vi "OAT Torsional Vibration (Digital Tacho) (Waveform) (1 Ch).vi"(0 "digital tacho info":T1={"tacho counts"=[], "counter timebase [Hz]"=1000.0, "counter task type"=enum."event counting", "counter digit (32)"=32}, 2 "pulse/revolution (1)":i32=1 min=1, 4 "torsional vibration units":enum16{"RPM", "deg/s", "rad/s"}(ring), 5 "error in (no error)":errorcluster, 8 "reset? (F)":bool, 10 "compensate geometric imperfection? (F)":bool, 11 "output interval [s]":dbl=0.001 min=0.0) -> (14 "torsional vibration signal":waveform(dbl), 15 "speed profile":T2 {"speed [RPM]" format="%.2f"; "time [s]" format="%.2f"}, 18 "unit label":string, 19 "error out":errorcluster)   [LabVIEW 2017, in "SoundVib_Torsional.lvlib"]
doc: "Calculates torsional vibration signals from digital tachometer signals. This VI can return torsional vibration signals as either waveform signals or even-angle signals. Wire data to the <B>digital tacho info</B> input to determine the polymorphic instance to use or manually select the instance."
uses:
  <vilib>/addons/Sound and Vibration/Order Analysis/Torsional Vibration/SoundVib_Torsional.lvlib
  <vilib>/addons/Sound and Vibration/Order Analysis/Tach Process/SubVIs/speed profile.ctl
  <vilib>/addons/Sound and Vibration/Order Analysis/Tach Process/SubVIs/digital tach info.ctl
  <vilib>/addons/Sound and Vibration/Order Analysis/Tach Process/SoundVib_TachProcess.lvlib
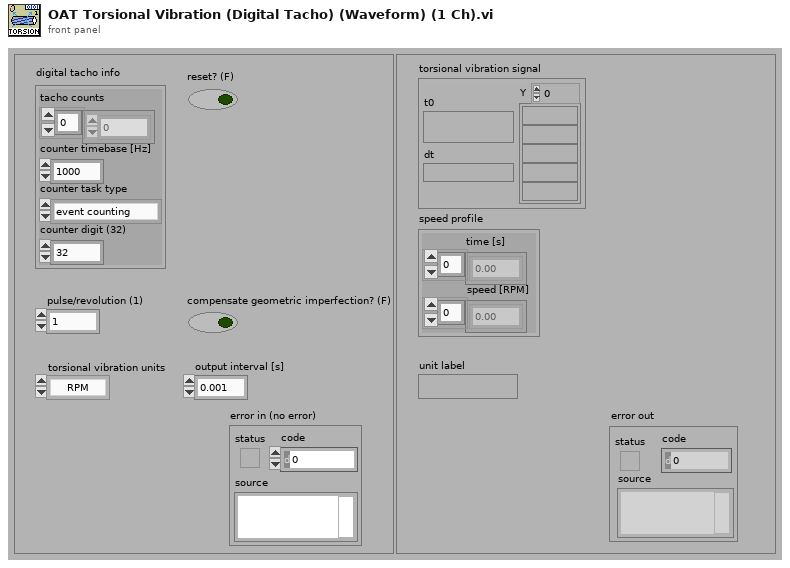
[diagram p1: front panel]
types:
  T1 = typedef "SoundVib_TachProcess.lvlib/digital tach info.ctl" = cluster{"tacho counts":i64[], "counter timebase [Hz]":dbl, "counter task type":enum16{"period measurement", "event counting"}, "counter digit (32)":i32}
  T2 = typedef "SoundVib_TachProcess.lvlib/speed profile.ctl" = cluster{"time [s]":dbl[], "speed [RPM]":dbl[]}
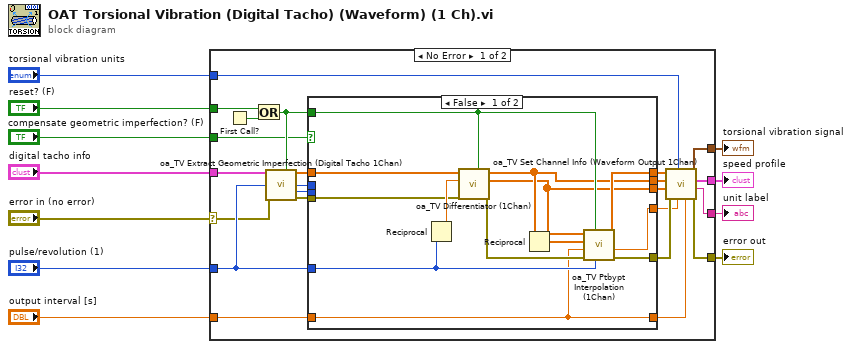
[diagram p0: block diagram]
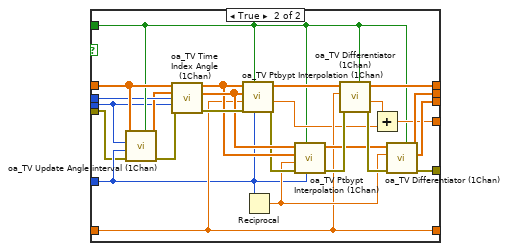
[diagram p2: hidden frame]
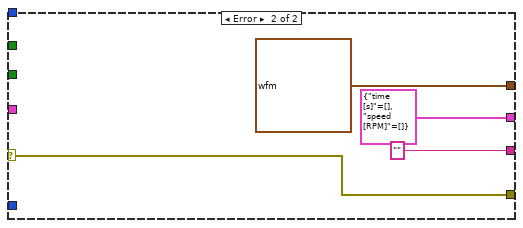
[diagram p3: hidden frame]
diagram:
  n1 = case shown="No Error" "error in (no error)" {
    selector: "error in (no error)" -> [w25 w75]
    tunnel: "pulse/revolution (1)" -> [w27 _]
    tunnel: [w20 waveform(dbl) {"t0"=timestamp(0 s since 1904-01-01), "dt"=1.0, "Y"=[]} ("even time speed")] -> w11
    tunnel: "compensate geometric imperfection? (F)" -> [w13 _]
    tunnel: "reset? (F)" -> [w31 _]
    tunnel: "digital tacho info" -> [w29 _]
    tunnel: "output interval [s]" -> [w18 _]
    tunnel: "torsional vibration units" -> [w19 _]
    tunnel: [w23 w75] -> w5
    tunnel: [w16 T2 {"time [s]"=[], "speed [RPM]"=[]} ("speed profile")] -> w4
    tunnel: [w12 "" ("unit label")] -> w1
    frame No Error {
      n2 = First Call?() -> (First Call?: T/F=w32:bool)
      n3 = Or(x=w31, y=w32) -> (x .or. y?=w26:bool)
      n4 = call <vilib>:"oa_TV Extract Geometric Imperfection (Digital Tacho 1Chan).vi"("digital tach info"=w29, "reset? (F)"=w26, "pulse/revolution"=w27, "error in (no error)"=w25) -> ("pulse positions"=w28:dbl[], "revulotion"=w30:i32, "revulotion index"=w33:i32, "error out"=w34:errorcluster)  [unwired: 8 in]
      n5 = case shown="False" w13 {
        tunnel: w34 -> [w45 w49]
        tunnel: w33 -> [_ w51]
        tunnel: w30 -> [_ w53]
        tunnel: w28 -> [w47 w55]
        tunnel: w27 -> [w43 w50]
        tunnel: w26 -> [w39 w54]
        tunnel: [w35 w65] -> w24
        tunnel: [w38 w64] -> w22
        tunnel: [w44 w63] -> w21
        tunnel: w18 -> [w41 w59]
        tunnel: [w36 w56] -> w17
        tunnel: [w37 w60] -> w15
        tunnel: [w41 w59] -> w14
        frame False {
          n6 = Reciprocal(x=w43) -> (1/x=w46:dbl)
          n7 = call <vilib>:"oa_TV Differentiator (1Chan).vi"("reset? (True)"=w39, "error in (no error)"=w45, "deltaX"=w46, "Y[n]"=w47) -> ("error out"=w42:errorcluster, "X[n]"=w37:dbl[], "dY[n]/dX[n]"=w38:dbl[])  [unwired: 4 in, 1 out]
          n8 = Reciprocal(x=w38) -> (1/x=w40:dbl[])
          n9 = call <vilib>:"oa_TV Ptbypt Interpolation (1Chan).vi"("buffer size"=w43, "reset? (F)"=w39, "error in (no error)"=w42, "dX"=w41, "Y"=w40, "X"=w37) -> ("error out"=w35:errorcluster, "X0"=w36:dbl, "resampled Y"=w44:dbl[])  [unwired: 2 in, 1 out]
        }
        frame True {
          n10 = call <vilib>:"oa_TV Update Angle interval (1Chan).vi"("reset? (F)"=w54, "error in (no error)"=w49, "pulse/revolution"=w50, "revulotion index"=w51, "pulse positions"=w55) -> ("error out"=w48:errorcluster, "angle intervals"=w52:dbl[])  [unwired: 5 in]
          n11 = call <vilib>:"oa_TV Time Index Angle (1Chan).vi"("pulse positions"=w55, "angle intervals"=w52, "revolution"=w53, "revolution index"=w51, "error in (no error)"=w48) -> ("pulse positions"=w69:dbl[], "angle"=w70:dbl[], "error out"=w72:errorcluster)  [unwired: 8 in]
          n12 = call <vilib>:"oa_TV Ptbypt Interpolation (1Chan).vi"("buffer size"=w50, "reset? (F)"=w54, "error in (no error)"=w72, "dX"=w59, "Y"=w70, "X"=w69) -> ("error out"=w68:errorcluster, "X0"=w58:dbl, "resampled Y"=w71:dbl[])  [unwired: 2 in, 1 out]
          n13 = Reciprocal(x=w50) -> (1/x=w62:dbl)
          n14 = call <vilib>:"oa_TV Ptbypt Interpolation (1Chan).vi"("buffer size"=w50, "reset? (F)"=w54, "error in (no error)"=w68, "dX"=w62, "Y"=w69, "X"=w70) -> ("error out"=w67:errorcluster, "resampled Y"=w61:dbl[])  [unwired: 2 in, 2 out]
          n15 = call <vilib>:"oa_TV Differentiator (1Chan).vi"("reset? (True)"=w54, "error in (no error)"=w67, "deltaX"=w59, "Y[n]"=w71) -> ("error out"=w66:errorcluster, "Delay"=w57:dbl, "dY[n]/dX[n]"=w63:dbl[])  [unwired: 4 in, 1 out]
          n16 = Add(x=w57, y=w58) -> (x+y=w56:dbl)
          n17 = call <vilib>:"oa_TV Differentiator (1Chan).vi"("reset? (True)"=w54, "error in (no error)"=w66, "deltaX"=w62, "Y[n]"=w61) -> ("error out"=w65:errorcluster, "X[n]"=w60:dbl[], "dY[n]/dX[n]"=w64:dbl[])  [unwired: 4 in, 1 out]
        }
      }
      n18 = call <vilib>:"oa_TV Set Channel Info (Waveform Output 1Chan).vi"("output interval [s]"=w14, "t0"=w17, "torisional vibration unit (RPM)"=w19, "error in (no error)"=w24, "pulse position"=w15, "seconds/rev"=w22, "revolutions/sec"=w21) -> ("error out"=w23:errorcluster, "unit label"=w12:string, "speed profile"=w16:T2, "torsional vibration"=w20:waveform(dbl))  [unwired: 1 in]
    }
    frame Error {
    }
  }
  "torsional vibration signal" <- w11
  "error out" <- w5
  "speed profile" <- w4
  "unit label" <- w1
